vi "Clear Hub.vi"(4 "timeout ms (25000)":i32=10, 6 "Bytes per sample":i32=4, 8 "error in (no error)":errorcluster, 9 "hub port":u64=2, 10 "Number of samples":u64=1, 11 "RP Instrument in":refnum<class "RP Instrument.lvclass">) -> (0 "error out":errorcluster, 1 "bytes read":i32, 2 "data out":string, 3 "RP Instrument out":refnum<class "RP Instrument.lvclass">)   [LabVIEW 2024, in "RP Instrument.lvclass"]
uses:
  RP Instrument.lvclass
  <vilib>/Utility/error.llb/Error Cluster From Error Code.vi
  <vilib>/ErrorRing/Error Ring.xnode
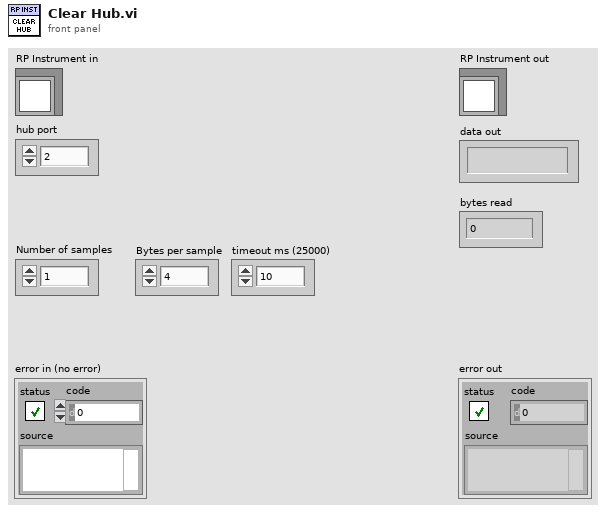
[diagram p1: front panel]
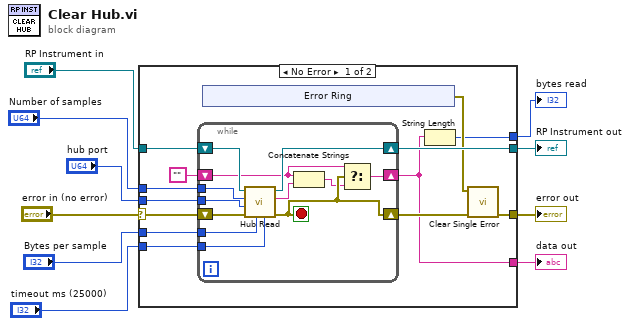
[diagram p0: block diagram]
diagram:
  n1 = case shown="No Error" "error in (no error)" {
    selector: "error in (no error)" -> [w21 w41]
    tunnel: [w15 w41] -> w9
    tunnel: [w23 w40] -> w7
    tunnel: "RP Instrument in" -> [w22 w40]
    tunnel: "hub port" -> [w20 _]
    tunnel: "timeout ms (25000)" -> [w19 _]
    tunnel: "Number of samples" -> [w18 _]
    tunnel: "Bytes per sample" -> [w17 _]
    tunnel: [w12 _] -> w2
    tunnel: [w11 _] -> w1
    frame No Error {
      n2 = while {
        tunnel: w20 -> [w37]
        shift-right: [w32] -> w23
        shift-left: w22 -> [w39]
        shift-right: [w31] -> w16
        shift-left: w21 -> [w38]
        tunnel: w19 -> [w36]
        tunnel: w18 -> [w35]
        tunnel: w17 -> [w34]
        shift-right: [w29] -> w12
        shift-left: "" -> [w30]
        stop <- w31 stop-if-true
        n3 = call-dynamic "Hub Read.vi"("timeout ms (25000)"=w36, "Bytes per sample"=w34, "error in (no error)"=w38, "hub port"=w37, "Number of samples"=w35, "RP Instrument in"=w39) -> ("error out"=w31:errorcluster, "data out"=w33:string, "RP Instrument out"=w32:refnum<class "RP Instrument.lvclass">)  [unwired: 3 in]
        n4 = Concatenate Strings(w30, w33) -> (w28:string)
        n5 = Select(t=w30, s=w31, f=w28) -> (s? t:f=w29:string)
      }
      n6 = xnode "Error Ring"() -> ("error out"=w14:errorcluster)
      n7 = String Length(string=w12) -> (length=w11:i32)
      n8 = call "Clear Single Error.vi"("Error In"=w16, "Error to clear"=w14) -> ("Error Out"=w15:errorcluster)  [unwired: 8 in, 1 out]
    }
    frame Error {
    }
  }
  "error out" <- w9
  "RP Instrument out" <- w7
  "data out" <- w2
  "bytes read" <- w1
